vi "UI Helper Loop Template.vi"   [LabVIEW 2019]
uses:
  <vilib>/ActorFramework/Actor/Actor.lvclass
  <vilib>/ActorFramework/Stop Msg/Stop Msg.lvclass
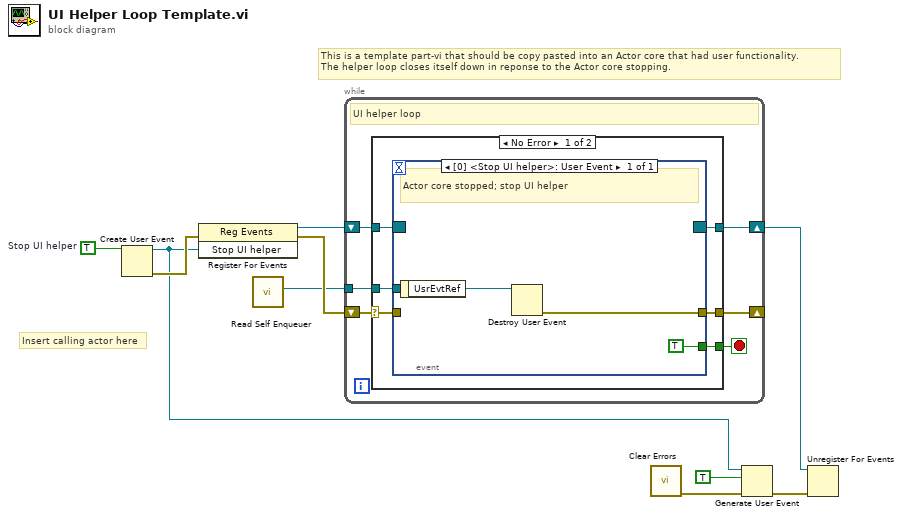
[diagram p0: block diagram]
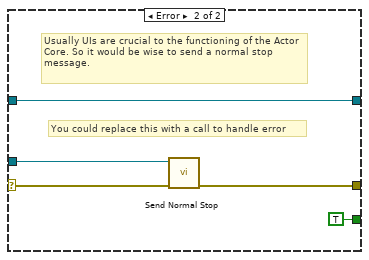
[diagram p2: hidden frame]
diagram:
  w9 = TRUE  # Stop UI helper
  # "Insert calling actor here"
  # "This is a template part-vi that should be copy pasted into an Actor core that had user functionality.\nThe helper loop closes itself down in reponse to the Actor core stopping."
  n1 = Create User Event(user event datatype=w9) -> (user event=w5:refnum<user-event>, error out=w8:errorcluster)  [unwired: 1 in]
  n2 = register-events(error in=w8, w5) -> (reference out=w10:refnum<event-registration>, error out=w2:errorcluster)  [unwired: 1 in]
  n3 = call <vilib>:"Read Self Enqueuer.vi"() -> ("Self Enqueuer"=w1:refnum<class "Message Enqueuer.lvclass">)  [unwired: 11 in]
  n4 = while {
    shift-right: [w15] -> w7
    shift-left: w10 -> [w16]
    shift-right: [w12] -> _
    shift-left: w2 -> [w13]
    tunnel: w1 -> [w11]
    stop <- w14 stop-if-true
    # "UI helper loop"
    n5 = case shown="No Error" w13 {
      selector: w13 -> [w19 w28]
      tunnel: w16 -> [w22 w30]
      tunnel: [w21 w30] -> w15
      tunnel: [w20 TRUE] -> w14
      tunnel: [w18 w27] -> w12
      tunnel: w11 -> [w17 w26]
      frame No Error {
        n6 = event shown="[0] <Stop UI helper>: User Event" {
          selector: w22 -> [_]
          dyn-events: [_] -> w21
          timeout: _ -> [_]
          tunnel: [TRUE] -> w20
          tunnel: w19 -> [_]
          tunnel: [w23] -> w18
          tunnel: w17 -> [_]
          event User Event {
            # "Actor core stopped; stop UI helper"
            n7 = event-data() -> ("UsrEvtRef"=w24:refnum<user-event>)  [unwired: 1 in]
            n8 = Destroy User Event(user event=w24) -> (error out=w23:errorcluster)  [unwired: 1 in]
          }
        }
      }
      frame Error {
        # "You could replace this with a call to handle error"
        # "Usually UIs are crucial to the functioning of the Actor Core. So it would be wise to send a normal stop message."
        n9 = call <vilib>:"Send Normal Stop.vi"("error in (no error)"=w28, "Message Enqueuer"=w26) -> ("error out"=w27:errorcluster)  [unwired: 9 in]
      }
    }
  }
  n10 = call <vilib>:"Clear Errors.vi"() -> ("error out"=w3:errorcluster)  [unwired: 6 in, 1 out]
  n11 = Generate User Event(user event=w5, event data cluster=TRUE ("event data"), error in=w3) -> (error out=w6:errorcluster)  [unwired: 1 in, 1 out]
  n12 = Unregister For Events(event registration refnum=w7, error in=w6) -> ()  [unwired: 1 out]
